vi "PH_uOPA_DelayController.PC set Width while Feedback.vi"(0 "VI in":refnum<vi>, 2 "Width while Feedback":dbl, 5 "error in (no error)":errorcluster) -> (14 "VI out":refnum<vi>, 19 "error out":errorcluster)   [LabVIEW 2014, in "PH_uOPA_DelayController.lvlib"]
uses:
  PH_uOPA_DelayController.lvlib
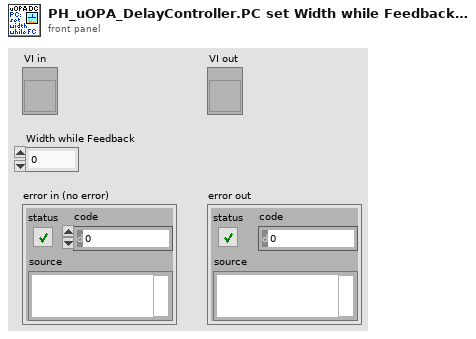
[diagram p1: front panel]
types:
  T1 = typedef "PH_uOPA_DelayController.lvlib/PH_uOPA_DelayController.i attribute.ctl" = cluster{"GUI Refs":cluster{"Current Pump Peak":refnum<vi>, "Current uOPA Peak":refnum<vi>, "Pump Peak":refnum<vi>, "uOPA Peak":refnum<vi>, "uOPA Target":refnum<vi>, "uOPA Limits [%]":refnum<vi>, "sample length":refnum<vi>, "Pump Target":refnum<vi>, "Pump Limit":refnum<vi>, "Pump running":refnum<vi>, "Feedback Control":refnum<vi>, "Control Status":refnum<vi>, "uOPA Mean":refnum<vi>, "Current uOPA Mean":refnum<vi>}, "uOPA Target":dbl, "uOPA Limits [%]":T2, "Sample Length":i32, "Initialize Mean":bool, "Pump Target":dbl, "Pump Limit [%]":dbl, "Feedback Control":bool, "Control Status":T3, "last Mean":dbl, "last direction":T4, "Axis Settings":T5, "Width while feedback":dbl}
  T2 = typedef "PH_uOPA_DelayController.lvlib/PH_uOPA_DelayController.Limit.ctl" = cluster{"low":dbl, "activate":dbl, "fine":dbl}
  T3 = typedef "PH_uOPA_DelayController.lvlib/PH_uOPA_DelayController.Control Status.ctl" = enum32{"off", "Pump off", "calculating", "too low", "activated", "fine"}
  T4 = typedef "PH_Stepmotor_BaseClass.lvlib/PH_Stepmotor_BaseClass.Axis Direction.ctl" = enum16{"forward", "backward"}
  T5 = typedef "PH_Stepmotor_BaseClass.lvlib/PH_Stepmotor_BaseClass.Axis Settings.ctl" = cluster{"Sign change":bool, "Width":dbl, "Calibration":dbl, "Unit":string, "Motor Type":T6, "Unit Width":string, "Unit CF":string}
  T6 = typedef "PH_Stepmotor_BaseClass.lvlib/PH_Stepmotor_BaseClass.Motor Type.ctl" = enum16{"Unspecific", "OWIS 49.120.2633", "OWIS 49.060.1033", "OWIS 43.040.2558", "Diamond Motion 2200 series", "OWIS 49.120.266B.MV6", "Calorimeter", "Linear Stage 1", "MICOS VT-80", "MICOS VT-80 S", "Standa Rotstage nt0.95A", "PUF RA 320.200", "PUF RA 800.200", "PUF RA 800.400", "PUF RA 400.50", "1324.nn.800.50", "1324.n9c.800.50", "1324.nn.320.200", "1324.nn.400.200", "1324.nn.800.200", "1324.nn.400.50", "1324.8c9c.800.50", "1324.8c9c.400.200"}
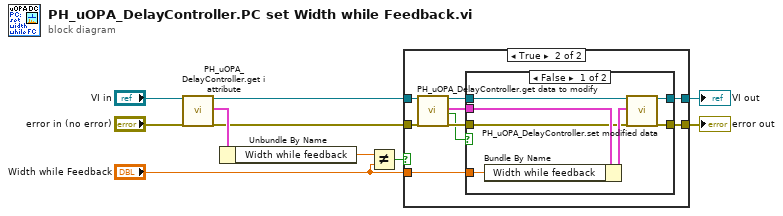
[diagram p0: block diagram]
diagram:
  n1 = call "PH_uOPA_DelayController.get i attribute.vi"("i ref in"="VI in", "error in (no error)"="error in (no error)") -> ("i ref out"=w6:refnum<vi>, "i attribute"=w7:T1, "error out"=w4:errorcluster)  [unwired: 15 in]
  n2 = Unbundle By Name(w7) -> ("Width while feedback"=w8:dbl)
  n3 = Not Equal?(x=w8, y="Width while Feedback") -> (x != y?=w10:bool)
  n4 = case shown="True" w10 {
    tunnel: [w11 w20] -> w2
    tunnel: [w12 w18] -> w3
    tunnel: w4 -> [w11 w15]
    tunnel: w6 -> [w12 w14]
    tunnel: "Width while Feedback" -> [_ w13]
    frame False {
    }
    frame True {
      n5 = call "PH_uOPA_DelayController.get data to modify.vi"("i ref in"=w14, "error in (no error)"=w15) -> ("i ref out"=w19:refnum<vi>, "i attribute"=w16:T1, "timed out"=w17:bool, "error out"=w21:errorcluster)  [unwired: 14 in]
      n6 = case shown="False" w17 {
        tunnel: w21 -> [w22 w29]
        tunnel: [w28 w29] -> w20
        tunnel: w19 -> [w27 w30]
        tunnel: [w26 w30] -> w18
        tunnel: w16 -> [w24 _]
        tunnel: w13 -> [w23 _]
        frame False {
          n7 = Bundle By Name(cluster=w24, "Width while feedback"=w23) -> (w25:T1)
          n8 = call "PH_uOPA_DelayController.set modified data.vi"("i ref in"=w27, "i attribute"=w25, "error in (no error)"=w22) -> ("i ref out"=w26:refnum<vi>, "error out"=w28:errorcluster)  [unwired: 15 in]
        }
        frame True {
        }
      }
    }
  }
  "VI out" <- w3
  "error out" <- w2
